vi "Dlg Open File.vi"(8 "error in":errorcluster, 11 "Log in":refnum<class "Log.lvclass">) -> (0 "error out":errorcluster, 2 "cancelled":bool, 3 "Log out":refnum<class "Log.lvclass">)   [LabVIEW 2017, in "Reports.lvlib" / "Log.lvclass"]
doc: "This Empty Dynamic basic method\nOpen Dialog window \nfor inheritance in child classes"
uses:
  Log.lvclass
  Log.lvclass/Log.ctl
panel:
  out "selected path":path
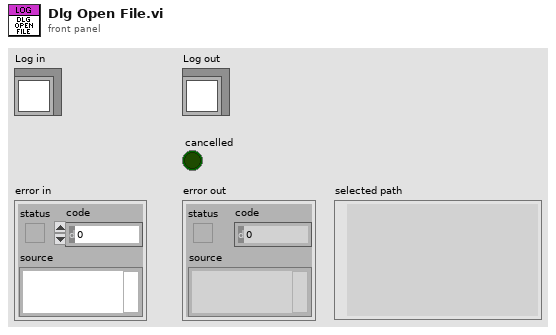
[diagram p1: front panel]
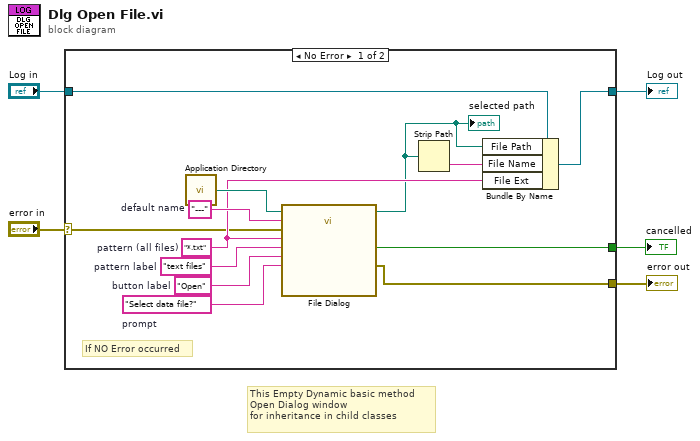
[diagram p0: block diagram]
diagram:
  # "This Empty Dynamic basic method\nOpen Dialog window \nfor inheritance in child classes"
  n1 = case shown="No Error" "error in" {
    selector: "error in" -> [w7 w20]
    tunnel: [w6 w20] -> w4
    tunnel: [w8 w19] -> w2
    tunnel: "Log in" -> [w9 w19]
    tunnel: [w10 _] -> w1
    frame No Error {
      w14 = "text files"  # pattern label
      w15 = "Select data file?"  # prompt
      w16 = "Open"  # button label
      w12 = "*.txt"  # pattern (all files)
      w17 = "---"  # default name
      # "If NO Error occurred"
      n2 = call <vilib>:"Application Directory.vi"() -> ("Application Directory"=w18:path)
      n3 = call "File Dialog"("start path"=w18, "prompt"=w15, "button label"=w16, "default name"=w17, "error in"=w7, "pattern (all files)"=w12, "pattern label"=w14) -> ("selected path"=w11:path, "cancelled"=w10:bool, "error out"=w6:errorcluster)  [unwired: 5 in, 1 out]
      "selected path" <- w11
      n4 = Strip Path(path=w11) -> (name=w13:string)  [unwired: 1 out]
      n5 = Bundle By Name(cluster=w9, "File Path"=w11, "File Name"=w13, "File Ext"=w12) -> (w8:refnum<class "Log.lvclass">)
    }
    frame Error {
    }
  }
  "error out" <- w4
  "Log out" <- w2
  "cancelled" <- w1
